vi "to_json.vi"(8 "error in":errorcluster, 11 "ts.logtime in":refnum<class "ts.logtime.lvclass">) -> (0 "error out":errorcluster, 2 "json":string, 3 "ts.logtime out":refnum<class "ts.logtime.lvclass">, 4 "Not Default":bool)   [LabVIEW 2020, in "ts.logtime.lvclass"]
uses:
  ts.logtime.lvclass
  <vilib>/JDP Science/JSONtext/Variant to JSON Text.vi
  <vilib>/JDP Science/JSONtext/LVClass Serializer/JSONtext LVClass Serializer.lvclass
  ts.logtime.lvclass/ts.logtime.ctl
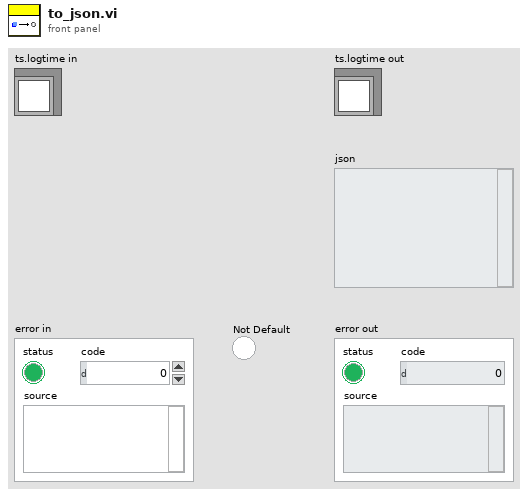
[diagram p1: front panel]
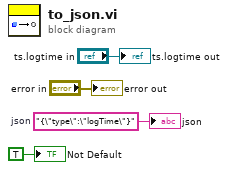
[diagram p0: block diagram]
diagram:
  w3 = "{\"type\":\"logTime\"}"  # json
  "ts.logtime out" <- "ts.logtime in"
  "error out" <- "error in"
  "json" <- w3
  "Not Default" <- TRUE ("Not Default")
